vi "ActiveObjects_QueueQueue_SendMsgToProcess_6x8x6_Singleton.vi"(1 "MessageToProcess":string, 5 "error in (no error)":errorcluster) -> (19 "error out":errorcluster)   [LabVIEW 2020]
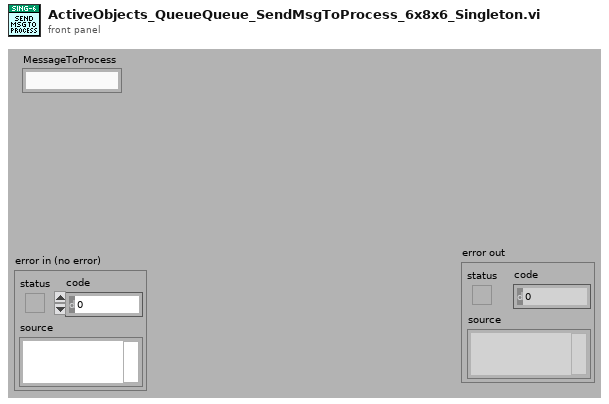
[diagram p1: front panel]
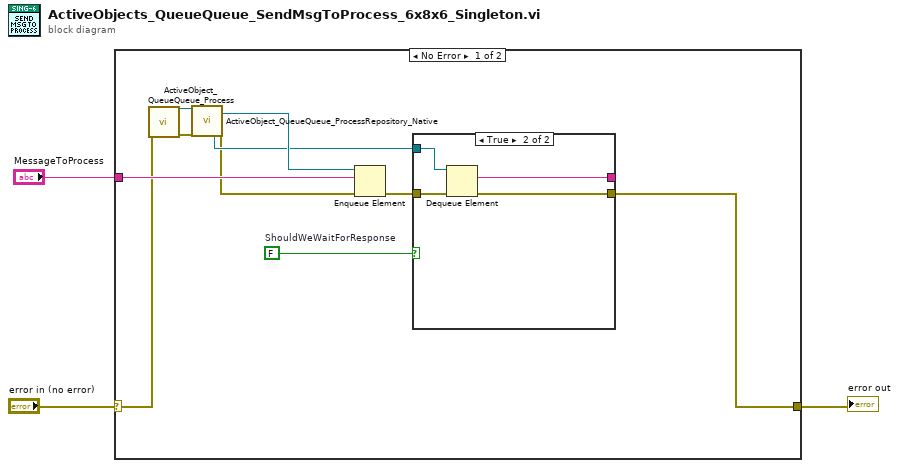
[diagram p0: block diagram]
diagram:
  n1 = case shown="No Error" "error in (no error)" {
    selector: "error in (no error)" -> [w5 w19]
    tunnel: [w7 w19] -> w2
    tunnel: "MessageToProcess" -> [w12 _]
    frame No Error {
      w11 = FALSE  # ShouldWeWaitForResponse
      n2 = call <resource>:"ActiveObject_QueueQueue_Process.vi"("error in (no error)"=w5) -> ("reference out"=w6:refnum<class>, "error out"=w4:errorcluster)  [unwired: 17 in]
      n3 = call <resource>:"ActiveObject_QueueQueue_ProcessRepository_Native.vi"("reference in"=w6, "error in (no error)"=w4) -> ("FromProcessQueue"=w9:refnum<queue>, "ToProcessQueue"=w13:refnum<queue>, "error out"=w8:errorcluster)  [unwired: 11 in, 4 out]
      n4 = Enqueue Element(queue=w13, element=w12, error in (no error)=w8) -> (error out=w10:errorcluster)  [unwired: 1 in, 2 out]
      n5 = case shown="True" w11 {
        tunnel: w10 -> [w14 w18]
        tunnel: w9 -> [_ w17]
        tunnel: [_ w16] -> _
        tunnel: [w14 w15] -> w7
        frame False {
        }
        frame True {
          n6 = Dequeue Element(queue=w17, error in (no error)=w18) -> (element=w16:string, error out=w15:errorcluster)  [unwired: 1 in, 2 out]
        }
      }
    }
    frame Error {
    }
  }
  "error out" <- w2
